vi "Actor Core.vi"(8 "error in":errorcluster, 11 "Sim Display Console Actor in":refnum<class "Sim Display Console Actor.lvclass">) -> (0 "error out":errorcluster, 3 "Actor out":refnum<class "Actor.lvclass">)   [LabVIEW 2022 SP3, in "Sim Display Console Actor.lvlib" / "Sim Display Console Actor.lvclass"]
doc: "(<B>Filename</B>: Actor Framework.lvlib:Actor.lvclass:Actor Core.vi)\n\nReceives messages to the actor, reacts to them, and initiates any error handling that may shut the actor down.\n\nDescendant classes may override this VI to append parallel tasks for the actor to complete while it handles messages. Overrides use the Call Parent Class Method node."
uses:
  Sim Display Console Actor.lvclass
  C:/Program Files/National Instruments/LabVIEW 2022/vi.lib/ActorFramework/Actor/Actor.lvclass
  <vilib>/ActorFramework/Actor/Actor.lvclass
  Sim Display Console Actor.lvclass/Sim Display Console Actor.ctl
  <vilib>/ActorFramework/Actor/Actor.lvclass/Actor.ctl
  <vilib>/ActorFramework/Message Enqueuer/Message Enqueuer.lvclass/Message Enqueuer.ctl
  <vilib>/ActorFramework/Message Enqueuer/Init from Existing Queue.vi
  <vilib>/ActorFramework/Message Enqueuer/Enqueue.vi
  <vilib>/ActorFramework/Stop Msg/Stop Msg.lvclass
  C:/Program Files/National Instruments/LabVIEW 2022/vi.lib/ActorFramework/Message/Message.lvclass
  <vilib>/ActorFramework/Message Priority Queue/Priority Enqueue.vi
  Abstract Display Console/Abstract Display Console/Abstract Display Console.lvclass
  <vilib>/ActorFramework/Message Enqueuer/Message Enqueuer.lvclass
panel:
  out "Elevator Direction":cluster{"Up":bool, "Down":bool}
  out "Emergency":bool
  out "Door open":bool
  out "Elevator Location":u32
  out "Timing":dbl
  # "[Covers: UI3C]"
  # "[Covers: UI3] \n[Covers: UI3A] \n[Covers: UI3A1] \n[Covers: UI3A2]"
  # "[Covers: UI3D]\n[Covers: UI3D1] \n[Covers: UI3D2]"
  # "[Covers: UI3B]"
  # "[Covers: UI3E]"
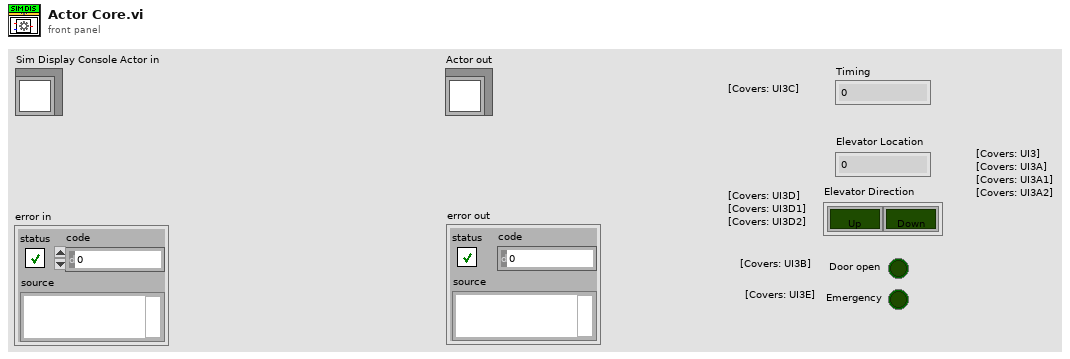
[diagram p1: front panel]
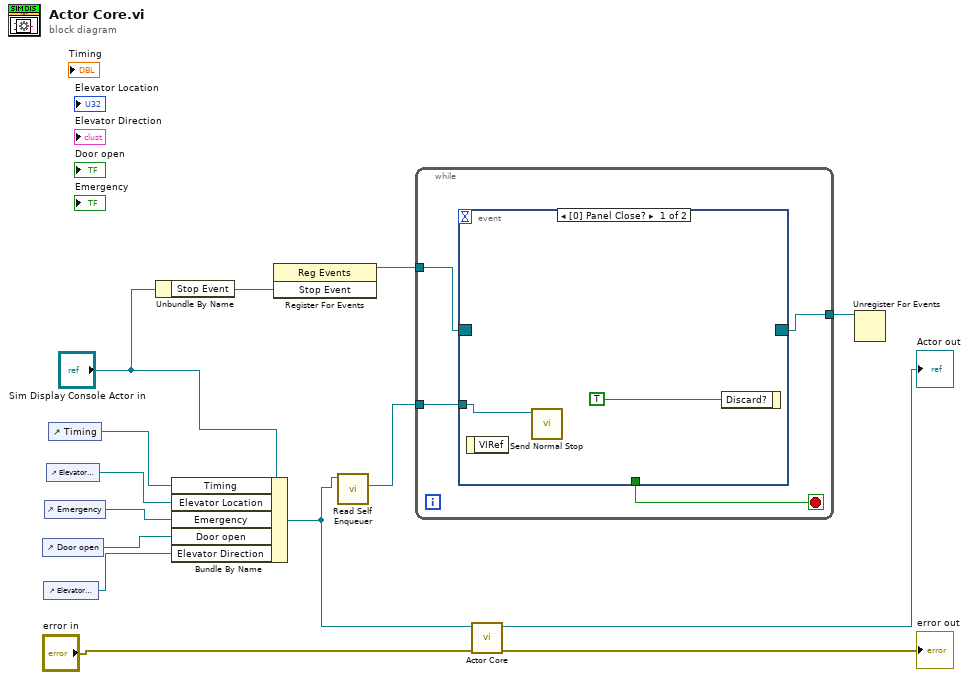
[diagram p0: block diagram]
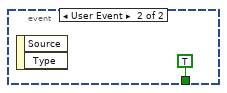
[diagram p2: hidden frame]
diagram:
  n1 = control-ref of="Door open"() -> (w8:refnum<vi>)
  n2 = control-ref of="Elevator Direction"() -> (w9:refnum<vi>)
  n3 = control-ref of="Emergency"() -> (w7:refnum<vi>)
  n4 = control-ref of="Elevator Location"() -> (w6:refnum<vi>)
  n5 = control-ref of="Timing"() -> (w5:refnum<vi>)
  n6 = Unbundle By Name("Sim Display Console Actor in") -> ("Stop Event"=w4:refnum<user-event>)
  n7 = Bundle By Name(cluster="Sim Display Console Actor in", "Timing"=w5, "Elevator Location"=w6, "Emergency"=w7, "Door open"=w8, "Elevator Direction"=w9) -> (w10:refnum<class "Sim Display Console Actor.lvclass">)
  n8 = register-events(w4) -> (reference out=w2:refnum<event-registration>)  [unwired: 2 in, 1 out]
  n9 = call <vilib>:"Read Self Enqueuer.vi"("Actor"=w10) -> ("Self Enqueuer"=w11:refnum<class "Message Enqueuer.lvclass">)  [unwired: 10 in]
  n10 = while {
    tunnel: w11 -> [w17]
    tunnel: w2 -> [w16]
    tunnel: [w15] -> w1
    stop <- w18 stop-if-true
    n11 = event shown="[0] Panel Close?" {
      selector: w16 -> [_ _]
      dyn-events: [_ _] -> w15
      timeout: _ -> [_ _]
      tunnel: [_ TRUE] -> w18
      tunnel: w17 -> [w19 _]
      event Panel Close? {
        n12 = event-data() -> ()  [unwired: 1 in, 1 out]
        n13 = call <vilib>:"Send Normal Stop.vi"("Message Enqueuer"=w19) -> ()  [unwired: 10 in, 1 out]
        n14 = event-data("Discard?"=TRUE) -> ()  [unwired: 1 in, 1 out]
      }
      event User Event {
        n15 = event-data() -> ()  [unwired: 1 in, 2 out]
      }
    }
  }
  n16 = call-parent "Actor Core.vi"("error in"="error in", "Actor in"=w10) -> ("error out"=→"error out":errorcluster, "Actor out"=→"Actor out":refnum<class "Actor.lvclass">)  [unwired: 8 in]
  n17 = Unregister For Events(event registration refnum=w1) -> ()  [unwired: 1 in, 1 out]
